vi "Split Ten 2 Five.vi"(0 "OUT 9:0":fxp<+,10,10> format="%08b") -> (4 "OUT 1:0":fxp<+,2,2>, 6 "OUT 1:0 2":fxp<+,2,2>, 8 "OUT 1:0 3":fxp<+,2,2>, 10 "OUT 1:0 4":fxp<+,2,2>, 15 "OUT 1:0 5":fxp<+,2,2>)   [LabVIEW 2019]
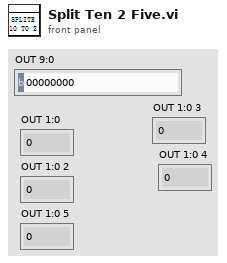
[diagram p1: front panel]
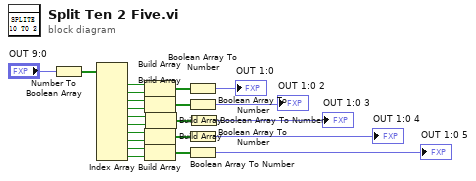
[diagram p0: block diagram]
diagram:
  n1 = Number To Boolean Array(number="OUT 9:0") -> (Boolean array=w21:bool[])
  n2 = Index Array(array=w21) -> (element #1=w19:bool, element #2=w18:bool, element #3=w16:bool, element #4=w15:bool, element #5=w13:bool, element #6=w9:bool, element #7=w11:bool, element #8=w8:bool, element #9=w7:bool, element #10=w6:bool)  [unwired: 10 in]
  n3 = Build Array(w19, w18) -> (w20:bool[])
  n4 = Build Array(w16, w15) -> (w17:bool[])
  n5 = Build Array(w11, w8) -> (w12:bool[])
  n6 = Build Array(w7, w6) -> (w10:bool[])
  n7 = Build Array(w13, w9) -> (w14:bool[])
  n8 = Boolean Array To Number(Boolean array=w20) -> (number=→"OUT 1:0":fxp<+,2,2>)
  n9 = Boolean Array To Number(Boolean array=w17) -> (number=→"OUT 1:0 2":fxp<+,2,2>)
  n10 = Boolean Array To Number(Boolean array=w12) -> (number=→"OUT 1:0 4":fxp<+,2,2>)
  n11 = Boolean Array To Number(Boolean array=w10) -> (number=→"OUT 1:0 5":fxp<+,2,2>)
  n12 = Boolean Array To Number(Boolean array=w14) -> (number=→"OUT 1:0 3":fxp<+,2,2>)
